vi "PolishVisionV3.vi"() -> ()   [LabVIEW 2015]
uses:
  <vilib>/userdefined/High Color/IMAQdx.ctl
  <vilib>/vision/NI_Vision_Development_Module.lvlib
  <vilib>/vision/driver/NI_Vision_Acquisition_Software.lvlib
panel:
  in  "stop":bool
  out "Matches (pixel)":T1(array[cluster]) {"Bounding Box"."y" format="%.2f"; "Bounding Box"."x" format="%.2f"; "Score" format="%.2f"; "Scale" format="%.2f"; "Angle" format="%.2f"; "Position"."y" format="%.2f"; "Position"."x" format="%.2f"}
  out "Image":T2(plugin-control)
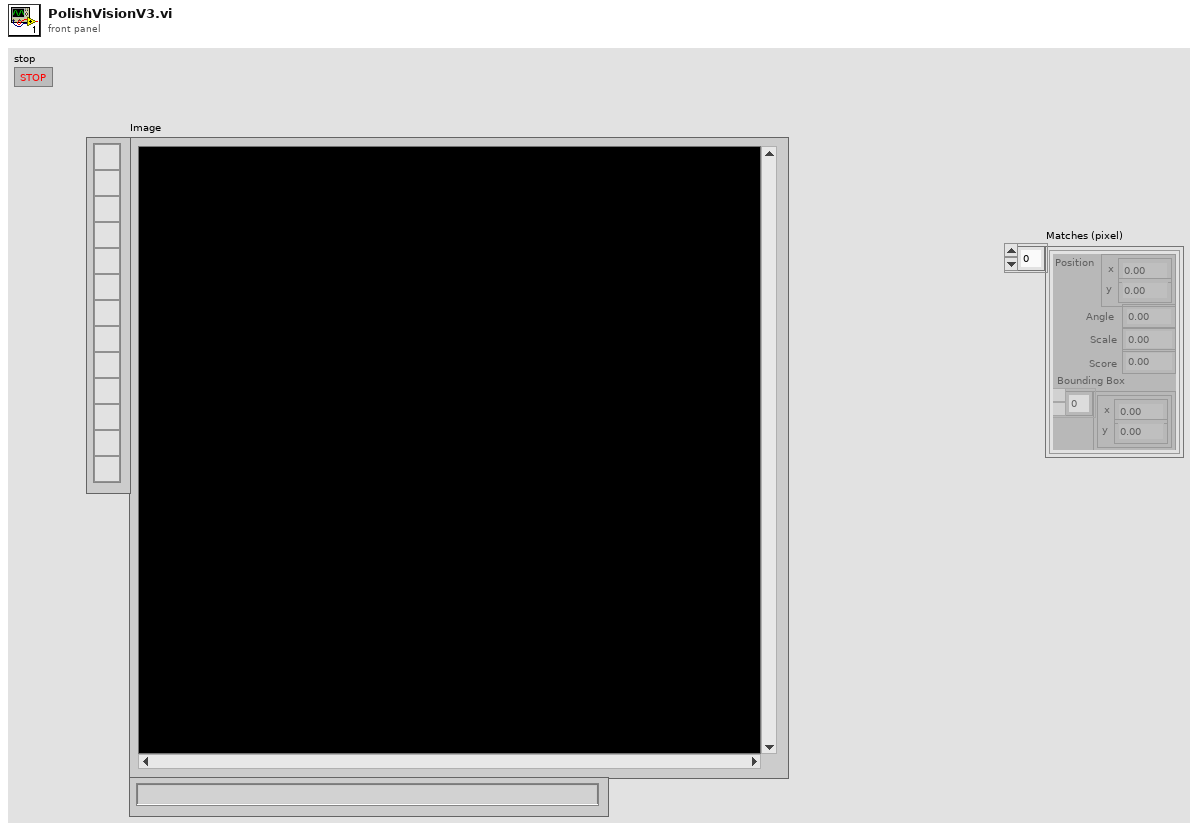
[diagram p1: front panel]
types:
  T1 = cluster{"Position":cluster{"x":sgl, "y":sgl}, "Angle":sgl, "Scale":sgl, "Score":sgl, "Bounding Box":cluster{"x":sgl, "y":sgl}[]}[]
  T2 = typedef "IMAQ Image.ctl" = refnum<image>
  T3 = cluster{"Global Rectangle":i32[], "Contours":cluster{"ID":enum32{"External", "Internal"}, "Type":u32, "Coordinates":i32[]}[]}
  T4 = cluster{"Number of Matches Requested":i32, "Minimum Match Score":sgl, "Angle Ranges":cluster{"Start Angle":sgl, "End Angle":sgl}[]}
  T5 = cluster{"Origin Pixel":cluster{"X":sgl, "Y":sgl}, "X Axis Pixel":cluster{"X":sgl, "Y":sgl}, "Axis Reference":u32}
  T6 = typedef "IMAQdx.ctl" = refnum<k21>
  T7 = typedef "Image Type" = u32
  T8 = cluster{"Feature":u32, "Points IDs":cluster{"GUID":string, "Index":i32}[]}[]
  T9 = cluster{"Matches (pixel)[0]":cluster{"Position":cluster{"x":sgl, "y":sgl}, "Angle":sgl, "Scale":sgl, "Score":sgl, "Bounding Box":cluster{"x":sgl, "y":sgl}[]}, "Matches (pixel)[1]":cluster{"Position":cluster{"x":sgl, "y":sgl}, "Angle":sgl, "Scale":sgl, "Score":sgl, "Bounding Box":cluster{"x":sgl, "y":sgl}[]}, "Matches (pixel)[2]":cluster{"Position":cluster{"x":sgl, "y":sgl}, "Angle":sgl, "Scale":sgl, "Score":sgl, "Bounding Box":cluster{"x":sgl, "y":sgl}[]}, "Matches (pixel)[3]":cluster{"Position":cluster{"x":sgl, "y":sgl}, "Angle":sgl, "Scale":sgl, "Score":sgl, "Bounding Box":cluster{"x":sgl, "y":sgl}[]}, "Matches (pixel)[4]":cluster{"Position":cluster{"x":sgl, "y":sgl}, "Angle":sgl, "Scale":sgl, "Score":sgl, "Bounding Box":cluster{"x":sgl, "y":sgl}[]}, "Matches (pixel)[5]":cluster{"Position":cluster{"x":sgl, "y":sgl}, "Angle":sgl, "Scale":sgl, "Score":sgl, "Bounding Box":cluster{"x":sgl, "y":sgl}[]}, "Matches (pixel)[6]":cluster{"Position":cluster{"x":sgl, "y":sgl}, "Angle":sgl, "Scale":sgl, "Score":sgl, "Bounding Box":cluster{"x":sgl, "y":sgl}[]}, "Matches (pixel)[7]":cluster{"Position":cluster{"x":sgl, "y":sgl}, "Angle":sgl, "Scale":sgl, "Score":sgl, "Bounding Box":cluster{"x":sgl, "y":sgl}[]}, "Matches (pixel)[8]":cluster{"Position":cluster{"x":sgl, "y":sgl}, "Angle":sgl, "Scale":sgl, "Score":sgl, "Bounding Box":cluster{"x":sgl, "y":sgl}[]}}
  T10 = cluster{"output string":sgl, "output string":sgl}
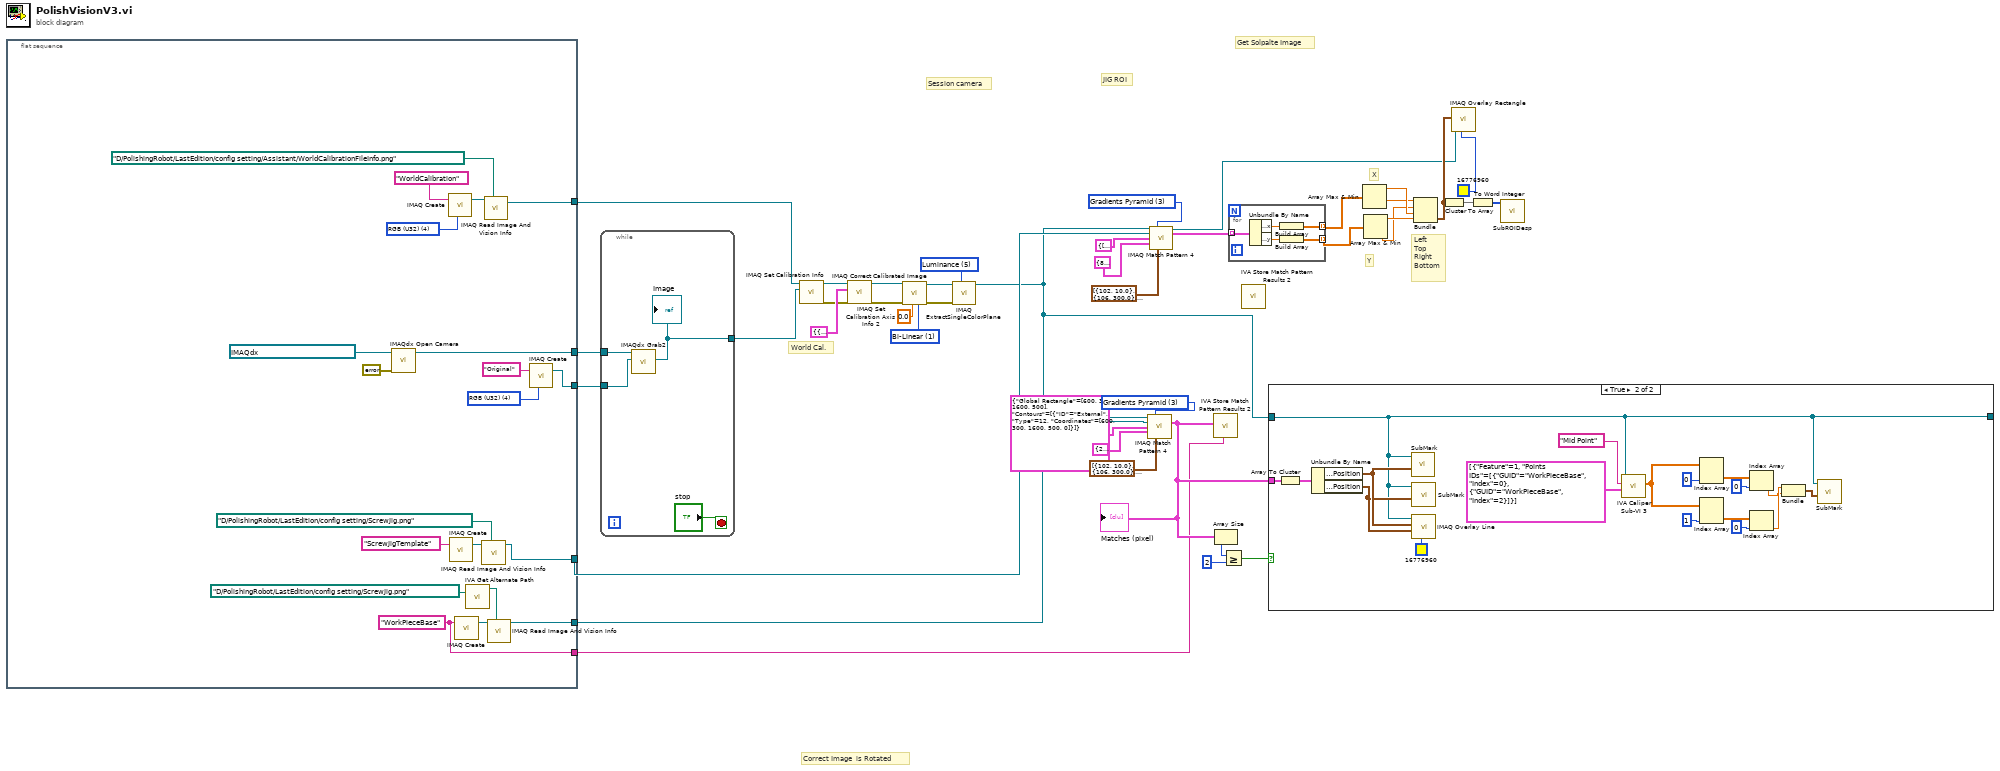
[diagram p0: block diagram]
diagram:
  w24 = 3 items=["All", "Low Discrepancy Sampling", "Grayscale Value Pyramid", "Gradients Pyramid"] ("Algorithm")
  w27 = 3 items=["All", "Low Discrepancy Sampling", "Grayscale Value Pyramid", "Gradients Pyramid"] ("Algorithm")
  w40 = u32 1 items=["Zero Order", "Bi-Linear", "Quadratic", "Cubic Spline"] ("Interpolation Type")
  w41 = 5 items=["Red", "Green", "Blue", "Hue", "Saturation", "Luminance", "Value", "Intensity"] ("Color Plane")
  # "Y"
  # "X"
  # "Left \nTop\nRight \nBottom"
  # "Correct Image  is Rotated"
  # "Session camera"
  # "World Cal."
  # "JIG ROI"
  # "Get Solpalte Image"
  n1 = flat-sequence {
    tunnel: [w59] -> w42
    tunnel: [w56] -> w15
    tunnel: [w49] -> w12
    tunnel: [w46] -> w11
    tunnel: [w44] -> w3
    tunnel: [w43] -> w2
    frame #0 {
      w62 = T7 4 items=["Grayscale (U8)", "Grayscale (I16)", "Grayscale (SGL)", "Complex (CSG)", "RGB (U32)", "HSL (U32)", "RGB (U64)", "Grayscale (U16)"] ("Image Type")
      w46 = "WorkPieceBase" ("Image Name")
      w52 = T7 4 items=["Grayscale (U8)", "Grayscale (I16)", "Grayscale (SGL)", "Complex (CSG)", "RGB (U32)", "HSL (U32)", "RGB (U64)", "Grayscale (U16)"] ("Image Type")
      n2 = call <vilib>:"IMAQdx Open Camera.vi"("error in"=errorcluster {"status"=FALSE, "code"=0, "source"=""}, "Session In"=T6 "RobotPolishCAM") -> ("Session Out"=w44:T6)  [unwired: 8 in, 1 out]
      n3 = call "IMAQ Create"("Image Name"="WorldCalibration", "Image Type"=w62) -> ("New Image"=w61:T2)  [unwired: 2 in, 2 out]
      n4 = call "IMAQ Create"("Image Name"="ScrewJigTemplate") -> ("New Image"=w58:T2)  [unwired: 3 in, 2 out]
      n5 = call "IMAQ Create"("Image Name"=w46) -> ("New Image"=w50:T2)  [unwired: 3 in, 2 out]
      n6 = call <vilib>:"IVA Get Alternate Path.vi"("Path In"=path "D:/PolishingRobot/LastEdition/config setting/ScrewJig.png" ("Template File Path")) -> ("Path Out"=w47:path)  [unwired: 10 out]
      n7 = call "IMAQ Read Image And Vision Info"("File Path"=path "D:/PolishingRobot/LastEdition/config setting/ScrewJig.png" ("Template File Path"), "Image"=w58) -> ("Image Out"=w56:T2)  [unwired: 2 in, 7 out]
      n8 = call "IMAQ Read Image And Vision Info"("File Path"=path "D:/PolishingRobot/LastEdition/config setting/Assistant/WorldCalibrationFileInfo.png", "Image"=w61) -> ("Image Out"=w59:T2)  [unwired: 2 in, 7 out]
      n9 = call "IMAQ Read Image And Vision Info"("File Path"=w47, "Image"=w50) -> ("Image Out"=w49:T2)  [unwired: 2 in, 7 out]
      n10 = call "IMAQ Create"("Image Name"="Original", "Image Type"=w52) -> ("New Image"=w43:T2)  [unwired: 3 in, 1 out]
    }
  }
  n11 = while {
    tunnel: w3 -> [w66]
    tunnel: w2 -> [w65]
    tunnel: [w63] -> w1
    stop <- "stop" stop-if-true
    n12 = call <vilib>:"IMAQdx Grab2.vi"("Image In"=w65, "Session In"=w66) -> ("Image Out"=w63:T2)  [unwired: 6 in, 3 out]
    "Image" <- w63
  }
  n13 = call "IMAQ Set Calibration Info"("Image Dst"=w1, "Image Src"=w42) -> ("error out"=w4:errorcluster, "Calibrated Image"=w10:T2)  [unwired: 2 in, 6 out]
  n14 = call-poly "IMAQ Set Calibration Axis Info 2"("error in (no error)"=w4, "Calibration Axis Info"=T5 {"Origin Pixel"={"X"=1112.4779, "Y"=2720.0552}, "X Axis Pixel"={"X"=1114.4336, "Y"=2720.047}, "Axis Reference"=0}, "Calibration Template Image In"=w10) -> ("error out"=w6:errorcluster, "Calibration Template Image Out"=w8:T2)  [unwired: 7 out]
  n15 = call "IMAQ Correct Calibrated Image"("Interpolation Type"=w40, "Replace Value"=sgl 0.0, "error in (no error)"=w6, "Image Src"=w8) -> ("error out"=w5:errorcluster, "Corrected Image"=w7:T2)  [unwired: 3 in, 3 out]
  n16 = call "IMAQ ExtractSingleColorPlane"("Color Plane"=w41, "error in (no error)"=w5, "Image Src"=w7) -> ("Image Dst Out"=w14:T2)  [unwired: 7 in, 1 out]
  n17 = call "IMAQ Match Pattern 4"("Image"=w14, "Algorithm"=w24, "Template Image"=w12, "ROI Descriptor"=T3 {"Global Rectangle"=[600, 300, 1600, 500], "Contours"=[{"ID"=enum."External", "Type"=12, "Coordinates"=[600, 300, 1600, 500, 0]}]}, "Parameters"=T4 {"Number of Matches Requested"=2, "Minimum Match Score"=500.0, "Angle Ranges"=[]}, "Advanced Options"=cluster{"Item":u16, "Value":dbl}[] [{"Item"=102, "Value"=10.0}, {"Item"=106, "Value"=300.0}, {"Item"=107, "Value"=0.0}, {"Item"=108, "Value"=6.0}, {"Item"=109, "Value"=1.0}, {"Item"=111, "Value"=20.0}, {"Item"=112, "Value"=10.0}, {"Item"=113, "Value"=20.0}, {"Item"=103, "Value"=1.0}, {"Item"=100, "Value"=1.0}]) -> ("Matches (pixel)"=w16:T1)  [unwired: 5 in, 4 out]
  "Matches (pixel)" <- w16
  n18 = call "IMAQ Match Pattern 4"("Image"=w14, "Algorithm"=w27, "Template Image"=w15, "ROI Descriptor"=T3 {"Global Rectangle"=[700, -20, 1533, 1079], "Contours"=[{"ID"=enum."External", "Type"=12, "Coordinates"=[700, -20, 1533, 1079, 0]}]}, "Parameters"=T4 {"Number of Matches Requested"=8, "Minimum Match Score"=500.0, "Angle Ranges"=[]}, "Advanced Options"=cluster{"Item":u16, "Value":dbl}[] [{"Item"=102, "Value"=10.0}, {"Item"=106, "Value"=300.0}, {"Item"=107, "Value"=0.0}, {"Item"=108, "Value"=6.0}, {"Item"=109, "Value"=1.0}, {"Item"=111, "Value"=20.0}, {"Item"=112, "Value"=10.0}, {"Item"=113, "Value"=20.0}, {"Item"=103, "Value"=1.0}, {"Item"=100, "Value"=1.0}]) -> ("Image (duplicate)"=w18:T2, "Matches (pixel)"=w13:T1)  [unwired: 5 in, 3 out]
  n19 = call <vilib>:"IVA Store Match Pattern Results 2.vi"("Step Name"=w11, "Matches (pixel)"=w16) -> ()  [unwired: 4 in, 6 out]
  n20 = Array Size(array=w16) -> (size(s)=w19:i32)
  n21 = Greater Or Equal?(x=w19, y=2) -> (x >= y?=w17:bool)
  n22 = for {
    tunnel: w13 -> [w71] mode=indexing
    tunnel: [w70] -> w37 mode=indexing
    tunnel: [w69] -> w38 mode=indexing
    n23 = Unbundle By Name(w71) -> ("Position.x"=w68:sgl, "Position.y"=w67:sgl)
    n24 = Build Array(w68) -> (w70:sgl[])
    n25 = Build Array(w67) -> (w69:sgl[])
  }
  n26 = call <vilib>:"IVA Store Match Pattern Results 2.vi"() -> ()  [unwired: 6 in, 6 out]
  n27 = case shown="True" w17 {
    tunnel: w16 -> [_ w89]
    tunnel: w14 -> [_ w74]
    tunnel: [_ w74] -> _
    frame False {
    }
    frame True {
      n28 = Array To Cluster(array=w89) -> (cluster=w88:T9)
      n29 = Unbundle By Name(w88) -> ("Matches (pixel)[0].Position"=w86:cluster{"x":sgl, "y":sgl}, "Matches (pixel)[1].Position"=w85:cluster{"x":sgl, "y":sgl})
      n30 = call "SubMark.vi"("Refnum in"=w74, "Position Pixel"=w86) -> ()  [unwired: 8 in]
      n31 = call "SubMark.vi"("Refnum in"=w74, "Position Pixel"=w85) -> ()  [unwired: 8 in]
      n32 = call "IMAQ Overlay Line"("Color"=u32 16776960, "End Point"=w85, "Start Point"=w86, "Image"=w74) -> ()  [unwired: 6 in, 2 out]
      n33 = call <vilib>:"IVA Caliper Sub-VI 3.vi"("Parameters"=T8 [{"Feature"=1, "Points IDs"=[{"GUID"="WorkPieceBase", "Index"=0}, {"GUID"="WorkPieceBase", "Index"=2}]}], "Step Name"="Mid Point", "Image In"=w74) -> ("Results (Pixels)"=w76:sgl[][])  [unwired: 2 in, 6 out]
      n34 = Index Array(array=w76, index (col)=0 ("disabled index (col)")) -> (element=w78:sgl[])  [unwired: 1 in]
      n35 = Index Array(array=w76, index (col)=1 ("disabled index (col)")) -> (element=w81:sgl[])  [unwired: 1 in]
      n36 = Index Array(array=w78, index=0) -> (element=w72:sgl)
      n37 = Index Array(array=w81, index=0) -> (element=w73:sgl)
      n38 = Bundle("output string"=w73, "output string"=w72) -> (w75:T10)  [unwired: 1 in]
      n39 = call "SubMark.vi"("Refnum in"=w74, "Position Pixel"=w75) -> ()  [unwired: 8 in]
    }
  }
  n40 = Array Max & Min(array=w37) -> (max value=w34:sgl, min value=w32:sgl)  [unwired: 2 out]
  n41 = Array Max & Min(array=w38) -> (max value=w35:sgl, min value=w33:sgl)  [unwired: 2 out]
  n42 = Bundle(w32, w33, w34, w35) -> (w25:cluster{sgl, sgl, sgl, sgl})  [unwired: 1 in]
  n43 = Cluster To Array(cluster=w25) -> (array=w36:sgl[])
  n44 = call "IMAQ Overlay Rectangle"("Color"=u32 16776960, "Rectangle"=w25, "Image"=w18) -> ()  [unwired: 7 in, 2 out]
  n45 = To Word Integer(number=w36) -> (16bit integer=w30:i16[])
  n46 = call "SubROIDesp.vi"("Array"=w30) -> ()  [unwired: 10 in, 1 out]
